vi "lab view graph and frequency.vi"() -> ()   [LabVIEW 2015]
panel:
  out "Waveform Chart":dynamicdata(graph)
  out "round frequency":dbl
  out "frequency":dbl
  in  "stop":bool
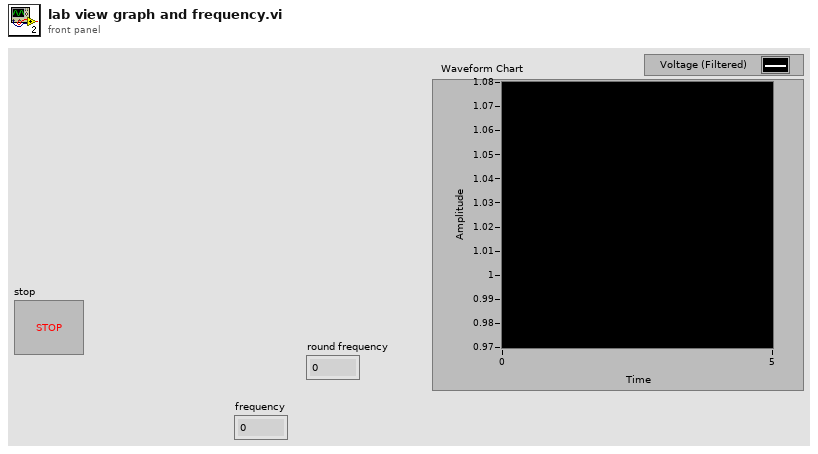
[diagram p1: front panel]
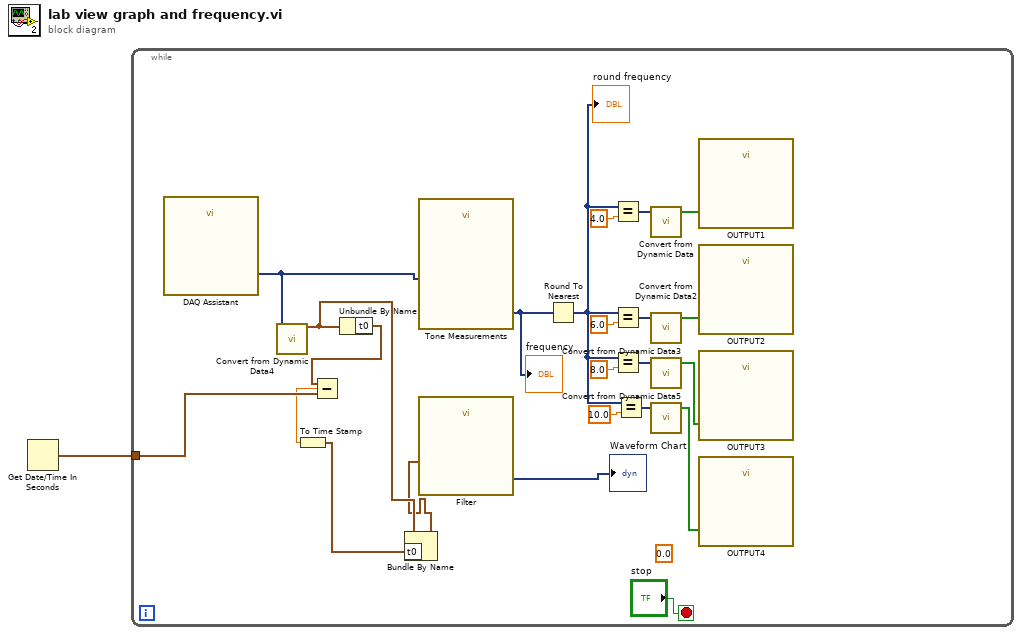
[diagram p0: block diagram]
diagram:
  n1 = Get Date/Time In Seconds() -> (seconds since 1Jan1904=w1:timestamp)
  n2 = while {
    tunnel: w1 -> [w9]
    stop <- "stop" stop-if-true
    (unwired) 0.0 ("y")
    n3 = call "DAQ Assistant"() -> ("data"=w7:dynamicdata)  [unwired: 16 in, 3 out]
    n4 = call "Convert from Dynamic Data4"("Dynamic Data Type"=w7) -> ("Waveform"=w4:waveform(dbl))  [unwired: 3 in]
    n5 = Unbundle By Name(w4) -> ("t0"=w6:timestamp)
    n6 = Subtract(x=w6, y=w9) -> (x-y=w8:dbl)
    n7 = To Time Stamp(1:w8) -> (0:w5:timestamp)
    n8 = Bundle By Name(cluster=w4, "t0"=w5) -> (w3:waveform(dbl))
    n9 = call "Tone Measurements"("Signals"=w7) -> ("Frequency"=w12:dynamicdata)  [unwired: 8 in, 2 out]
    "frequency" <- w12
    n10 = call "Filter"("Signal"=w3) -> ("Filtered Signal"=→"Waveform Chart":dynamicdata)  [unwired: 9 in, 1 out]
    n11 = Round To Nearest(number=w12) -> (nearest integer value=w11:dynamicdata)
    "round frequency" <- w11
    n12 = Equal?(x=w11, y=4.0) -> (x = y?=w15:dynamicdata)
    n13 = Equal?(x=w11, y=6.0) -> (x = y?=w19:dynamicdata)
    n14 = Equal?(x=w11, y=8.0) -> (x = y?=w17:dynamicdata)
    n15 = Equal?(x=w11, y=10.0) -> (x = y?=w10:dynamicdata)
    n16 = call "Convert from Dynamic Data"("Dynamic Data Type"=w15) -> ("Array"=w14:bool[])  [unwired: 3 in]
    n17 = call "Convert from Dynamic Data2"("Dynamic Data Type"=w19) -> ("Array"=w18:bool[])  [unwired: 3 in]
    n18 = call "Convert from Dynamic Data3"("Dynamic Data Type"=w17) -> ("Array"=w16:bool[])  [unwired: 3 in]
    n19 = call "Convert from Dynamic Data5"("Dynamic Data Type"=w10) -> ("Array"=w13:bool[])  [unwired: 3 in]
    n20 = call "OUTPUT1"("data"=w14) -> ()  [unwired: 17 in, 2 out]
    n21 = call "OUTPUT2"("data"=w18) -> ()  [unwired: 17 in, 2 out]
    n22 = call "OUTPUT3"("data"=w16) -> ()  [unwired: 17 in, 2 out]
    n23 = call "OUTPUT4"("data"=w13) -> ()  [unwired: 17 in, 2 out]
  }
